vi "OCT OpenCL.vi"() -> ()   [LabVIEW 2014]
doc: "I. Description:\nThis example demonstrates how to acquire a continuous amount of data (Waveform) using the DAQ device's internal clock.\n\nII. Instructions for Running:\n1. Create an analog input voltage channel.\n2. Set the rate for the sample clock. Additionally, define the sample mode to be continuous.\n3. Call the Start VI to start the acquisition.\n4. Read the waveform data in a loop until the user hits the stop button or an error occurs.\nNote: This example reads data from one or more channels and returns an array of data. Use the Index Array function to access an individual channel of data.\n5. Call the Clear Task VI to clear the Task.\n6. Use the popup dialog box to display an error if any.\n\nIV. I/O Connections Overview:\nMake sure your signal input terminal matches the Physical Channel I/O Control. For further connection information, refer to your hardware reference manual."
uses:
  ATS-VI/ATS_ctl/Device_Ctrl.ctl
  ATS-VI/ATS_ctl/ATS_Async_Ctrl.ctl
  ATS-VI/ATS_ctl/ATS_Async_Mode.ctl
  ATS-VI/ATS_ctl/ATS_DMA_Channel.ctl
  ATS-VI/ATS_ctl/ATS_ReadSamples.ctl
  ATS-VI/ATS_ctl/ATS_Check_Ctrl.ctl
  ATS-VI/ATS_ctl/ClockSource.ctl
  Galvo VIs/galvo_states.ctl
  Signal Processing/processing_states.ctl
  En Face/En Face States.ctl
  Saving Data/Saving Data States.ctl
  Type Defs/OCT Hardware States.ctl
  ATS-VI/ATS_ctl/Range.ctl
  ATS-VI/ATS_ctl/Impedance.ctl
  Type Defs/OCT Imaging Parameters Cluster.ctl
  Signal Processing/Display Raw Data states.ctl
  ATS-VI/ATS_ctl/Record.ctl
  ATS-VI/ATS_ctl/ClockRate.ctl
  ATS-VI/ATS_ctl/ClockEdge.ctl
  ATS-VI/ATS_ctl/Clock.ctl
  ATS-VI/ATS_ctl/Coupling.ctl
  ATS-VI/ATS_ctl/Bandwidth.ctl
  ATS-VI/ATS_ctl/InputCtrl.ctl
  ATS-VI/ATS_ctl/TriggerOperation.ctl
  ATS-VI/ATS_ctl/TriggerEngine.ctl
  ATS-VI/ATS_ctl/ExtTrigRange.ctl
  ATS-VI/ATS_ctl/ExtTrigger.ctl
  ATS-VI/ATS_ctl/Trigger.ctl
  ATS-VI/ATS_ctl/ATS_Global.ctl
  OpenCL/OpenCL States.ctl
  <vilib>/RaptorView/OpenCLV/User Controls/Array Dimensions.ctl
  DAQ Status States.ctl
  Type Defs/Display States.ctl
  ATS-VI/ATS_ctl/ATS_Async_Setting.ctl
  Type Defs/OCT DAQ Channel Data Type.ctl
panel:
  out "Background Array":u16[](array[numeric])
  in  "Calibrate":bool
  in  "Save Sweep Button":bool
  in  "Linear?":bool
  in  "Data Format":T1
  out "BScan":sgl[][](graph)
  in  "Display":T2
  in  "Save Sweep":bool
  in  "Stop Button":bool
  in  "B-Scans Per Buffer":i32=1
  out "Current State":T3
  in  "Channels":tag="Dev2/ao0:1"
  in  "Trigger Source":tag="/Dev2/PFI7"
  in  "Imaging Parameters":T4={"Points Per A-Scan"=0, "A-Scans per B-Scan"=0, "Voltage Range"=1.0, "Card Resolution (bits)"=12}
  out "First Time?":bool=TRUE
  out "Save Data":bool
  in  "Async_Setting":T5
  out "Processing Finished":bool
  in  "OCT Hardware States":T3=enum."Initialize DAQ"
  out "Save State":T6=enum."Do Nothing"
  out "Clock Length":u32=9184
  out "Reset DAQ":bool
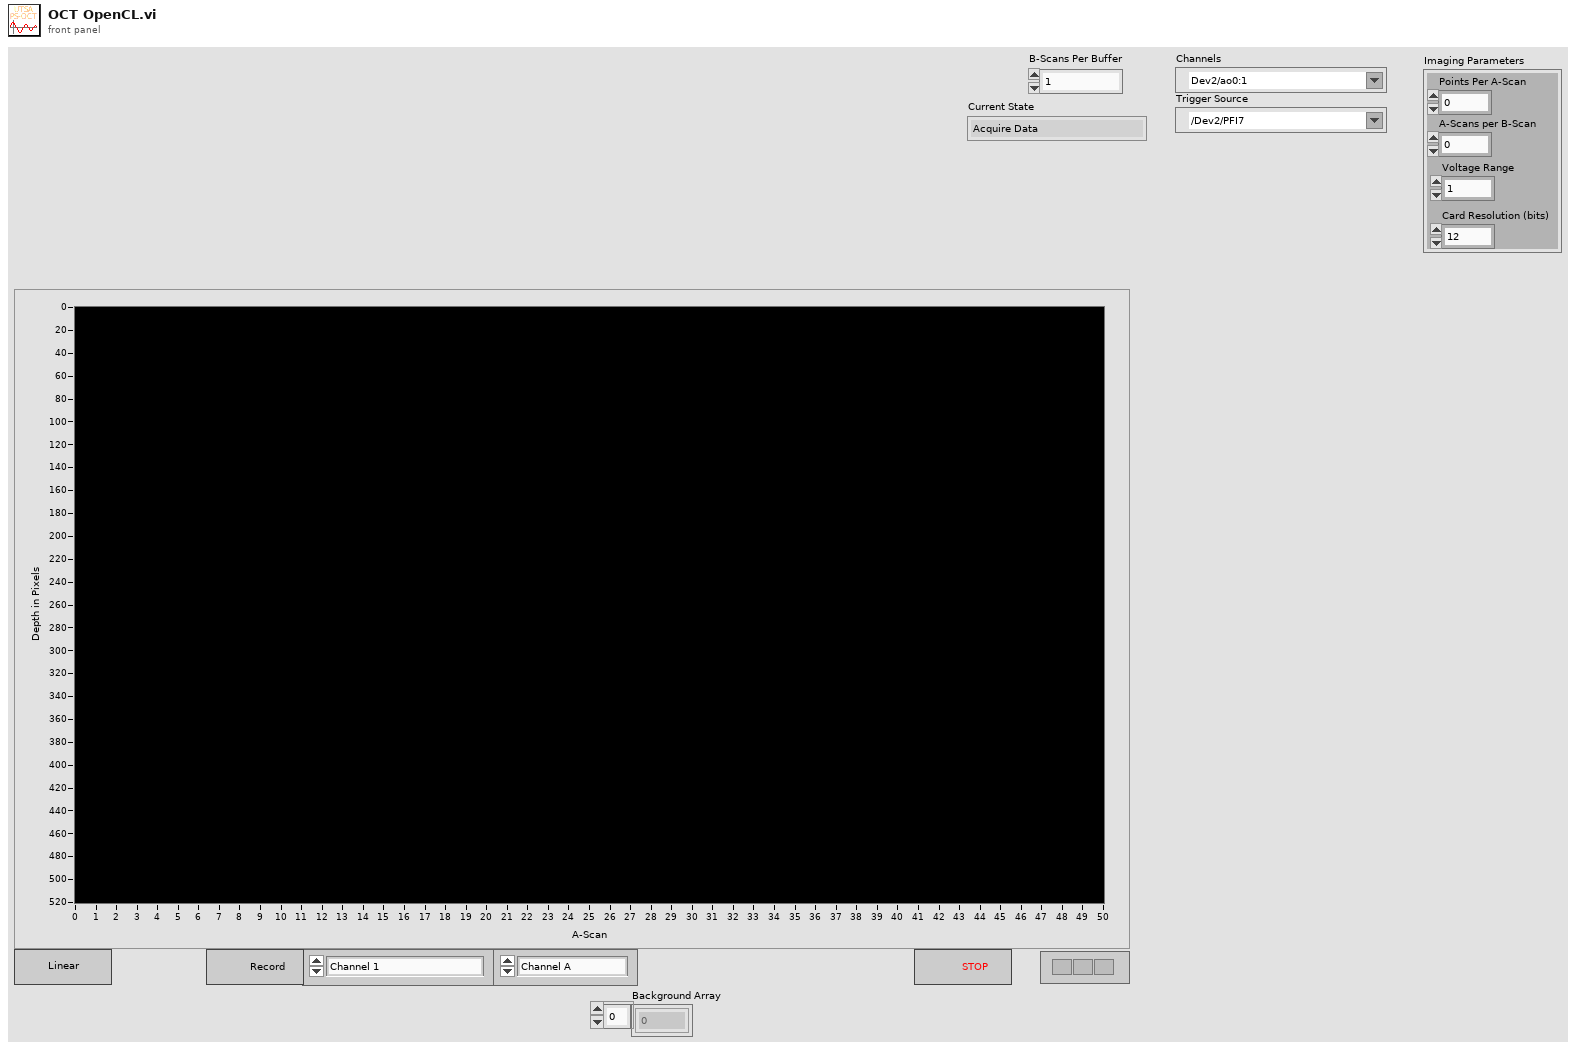
[diagram p1: front panel]
types:
  T1 = typedef "OCT DAQ Channel Data Type.ctl" = enum16{"Channel 1", "Channel 2", "Channel 1 and 2"}
  T2 = typedef "Display States.ctl" = enum16{"Channel A", "Channel B"}
  T3 = typedef "OCT Hardware States.ctl" = enum16{"Acquire Data", "Initialize Laser", "Initialize Galvos", "Startup", "Reset DAQ", "Background Subtraction", "Acquire Background", "Update DAQ Parameters", "Stop", "Set Clock", "Initialize DAQ", "Set Resampling Array", "Save Sweep", "Configure Laser"}
  T4 = typedef "OCT Imaging Parameters Cluster.ctl" = cluster{"Points Per A-Scan":i32, "A-Scans per B-Scan":i32, "Voltage Range":sgl, "Card Resolution (bits)":u16}
  T5 = typedef "ATS_Async_Setting.ctl" = cluster{"UseHeader":u32, "Rec/Buffer":u32, "Total_Rec":u32, "DataBuffer":bool, "GetProcessedData":bool}
  T6 = typedef "Saving Data States.ctl" = enum16{"Get Queue Size", "Get Queue", "Get Timeout", "Flush Queue", "Close Files", "Create Files", "Do Nothing", "Initialize", "Enqueue Data", "Save Data", "Shutdown"}
  T7 = typedef "ATS_Global.ctl" = cluster{"Record":T8, "Clock":T9, "Input A":T13, "Input B":T13, "Trigger":T18}
  T8 = typedef "Record.ctl" = cluster{"Count":u32, "Presize":u32, "Length":u32}
  T9 = typedef "Clock.ctl" = cluster{"ClckSource":T10, "ClckRate":T11, "ClckEdge":T12, "Decimation":u32}
  T10 = typedef "ClockSource.ctl" = enum16{"Internal", "External", "Medium Ext.", "Slow Ext.", "Ext. AC", "Ext. DC", "Ext. (PLL)"}
  T11 = typedef "ClockRate.ctl" = u32
  T12 = typedef "ClockEdge.ctl" = u16
  T13 = typedef "InputCtrl.ctl" = cluster{"Coupling":T14, "Range":T15, "Impedance":T16, "Bandwidth":T17}
  T14 = typedef "Coupling.ctl" = enum16{"AC", "DC"}
  T15 = typedef "Range.ctl" = u32
  T16 = typedef "Impedance.ctl" = enum16{"1M ohms", "50 ohms"}
  T17 = typedef "Bandwidth.ctl" = enum16{"Full Bandwidth", "Reduce Bandwidth"}
  T18 = typedef "Trigger.ctl" = cluster{"TrigOperation":T19, "Timeout (s)":dbl, "Trig. Delay":u32, "Engine X":T20, "Engine Y":T20, "ExtTrigControl":T21}
  T19 = typedef "TriggerOperation.ctl" = enum16{"Only X", "Only Y", "X or Y", "X and Y", "X xor Y", "X and not Y", "not X and Y"}
  T20 = typedef "TriggerEngine.ctl" = cluster{"Source":enum32{"Chan_A", "Chan_B", "External", "Disable"}, "Slope":enum32{"Positive", "Negative"}, "Level":u32}
  T21 = typedef "ExtTrigger.ctl" = cluster{"Coupling":T14, "Range":T22}
  T22 = typedef "ExtTrigRange.ctl" = enum16{"1 V", "5 V", "TTL"}
  T23 = typedef "galvo_states.ctl" = enum16{"Reset", "Reset Galvos?", "Center Galvos", "Register Callback", "Get Scan Parameters", "Show", "Initialize", "Run Raster", "Load Raster", "Run Circle", "Shutdown"}
  T24 = typedef "OpenCL States.ctl" = enum16{"Allocate Memory", "Get U16 Memory Dimension", "Compile Kernels", "Create Device", "Write", "Read", "Operate", "Delete Memory", "Delete"}
  T25 = typedef "processing_states.ctl" = enum16{"Initialize", "Set Background", "Update Imaging Parameters", "Get Queue", "Process Data", "Get Size", "Flush Data", "Set Reample Array", "Get Last Processed BScan", "Shutdown"}
  T26 = typedef "En Face States.ctl" = enum16{"Save BMP", "Show", "Clear En Face", "Update EnFace"}
  T27 = typedef "Galvo.lvclass/Scanning Cluster.ctl" = cluster{"Fast Axis Offset":sgl, "Slow Axis Offset":sgl, "Slow Axis Amp":sgl, "Fast Axis Amp":sgl, "Scan Pattern":enum16{"Raster"}}
  T28 = typedef "Processed OCT Data.ctl" = cluster{"Intensity A":sgl[][][], "Intensity B":sgl[][][]}
  T29 = typedef "ATS_Async_Ctrl.ctl" = enum16{"SetupDMA", "StartCapture", "Get", "Get_Stream", "Abort", "Stop"}
  T30 = typedef "ATS_ReadSamples.ctl" = cluster{"Offset":i32, "Length":u32}
  T31 = typedef "ATS_DMA_Channel.ctl" = enum16{"Channel_A", "Channel_B", "A & B"}
  T32 = typedef "ATS_Async_Mode.ctl" = enum16{"Continuous", "Triggered", "No-Pre-Trigger", "Traditional"}
  T33 = typedef "ATS_Check_Ctrl.ctl" = enum16{"None", "NO_ATS9462", "ATS9462_Traditional", "Verify Board", "OnBoard Memory", "Board & Memory", "Master/Slave", "NO Master/Slave"}
  T34 = typedef "Device_Ctrl.ctl" = enum16{"Status", "About", "Arm", "ForceTrig", "Abort", "Initialize", "Init (NoPreset)", "Info", "Close", "Calibrate", "SetManually", "LED_ON", "LED_OFF"}
  T35 = typedef "DAQ Status States.ctl" = enum16{"Get", "Show"}
  T36 = typedef "Display Raw Data states.ctl" = enum16{"Add Raw", "Add Processed", "Show"}
  T37 = typedef "Array Dimensions.ctl" = cluster{"Depth":u64, "Height":u64, "Width":u64}
  T38 = typedef "ATS_Async_Status.ctl" = cluster{"Start DMA":bool, "StartCapture":bool, "Valid":bool, "Completed":bool, "InProgress":bool, "Timeout":bool, "Overflow":bool, "Error":bool}
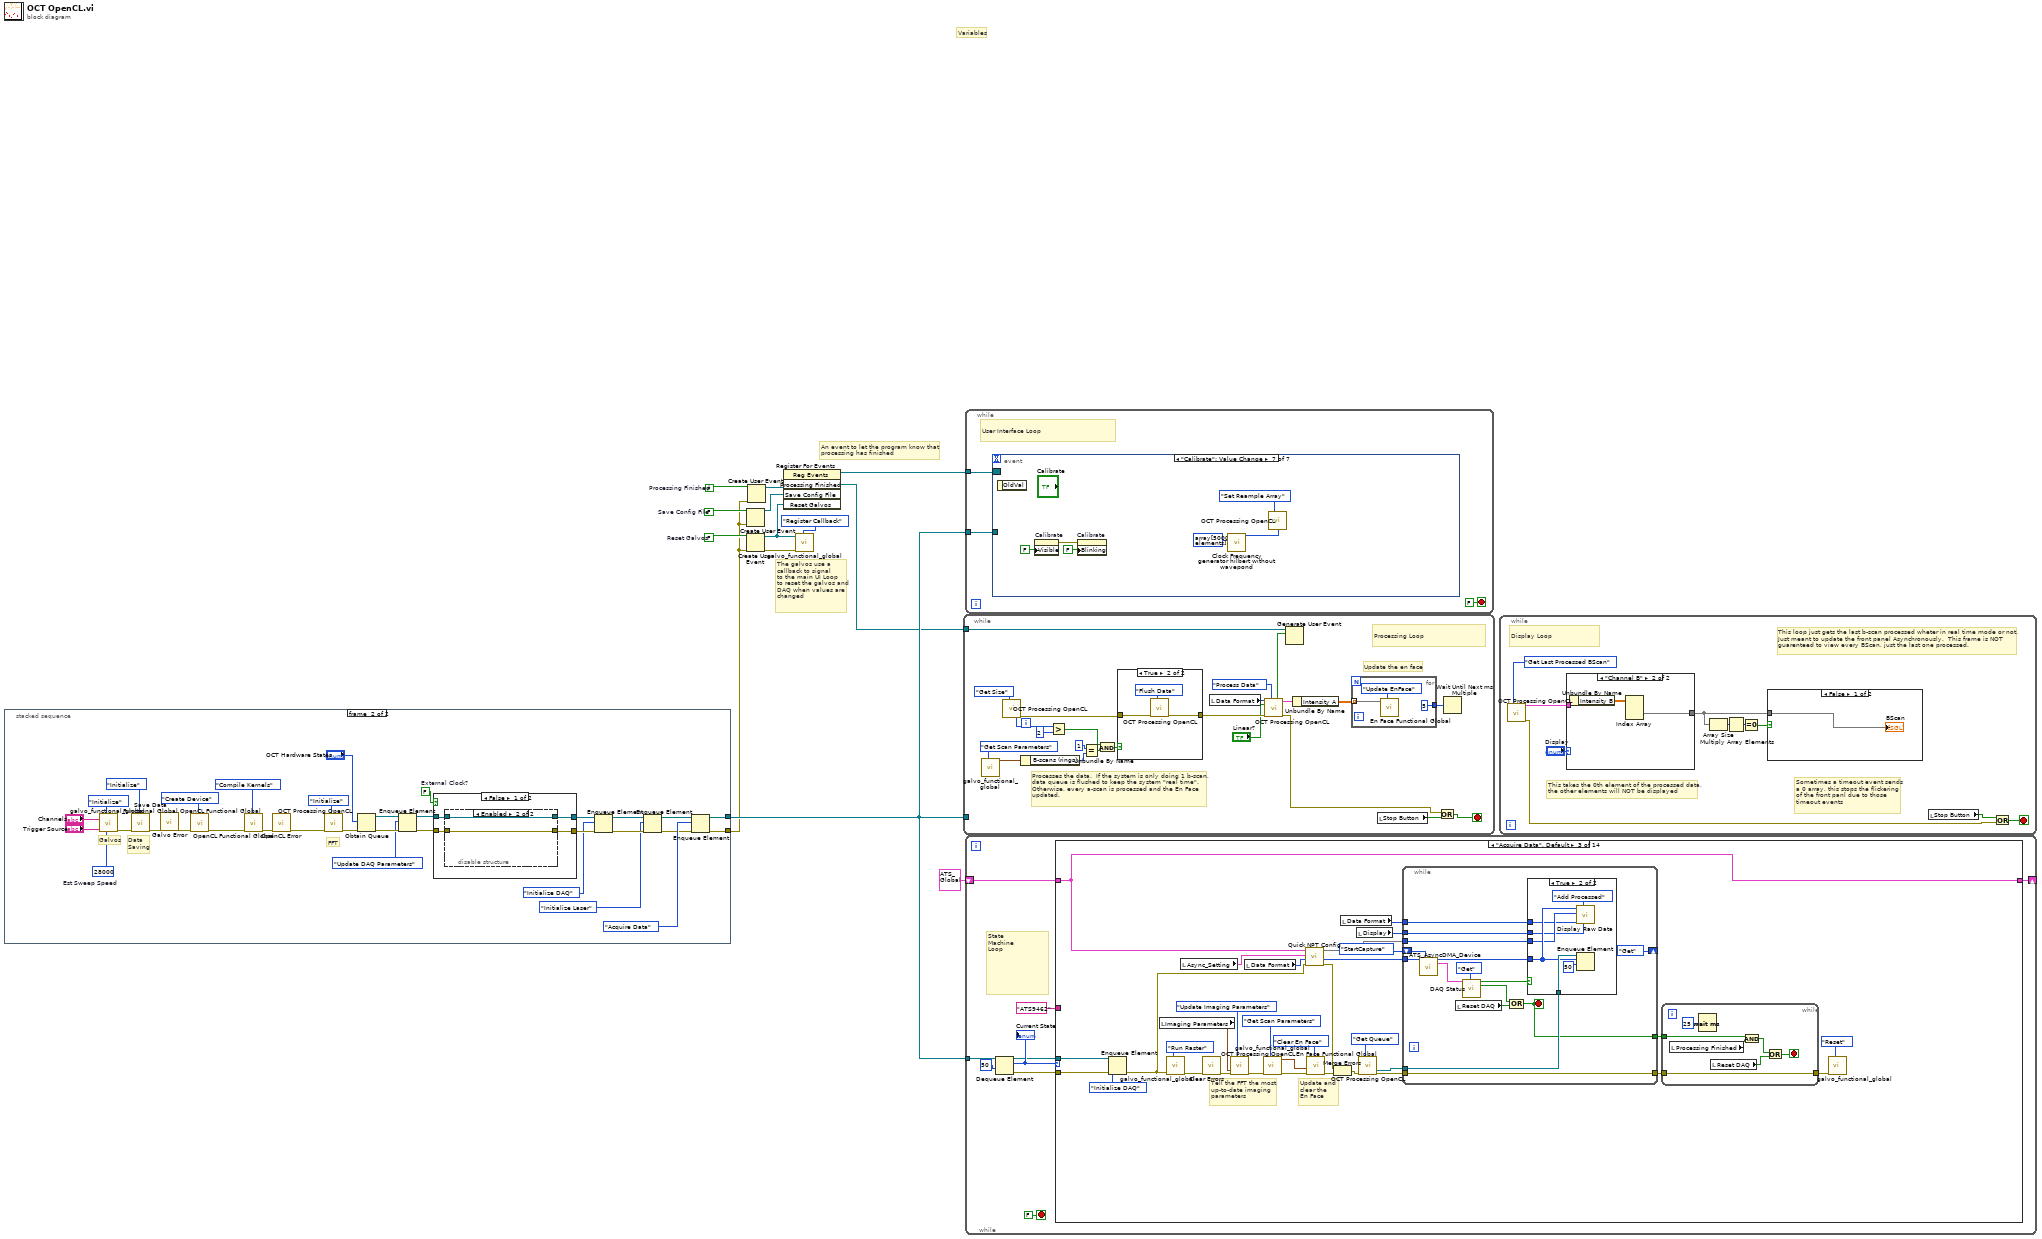
[diagram p0: block diagram]
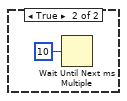
[diagram p3: hidden frame]
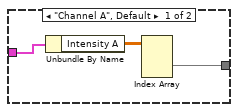
[diagram p4: hidden frame]
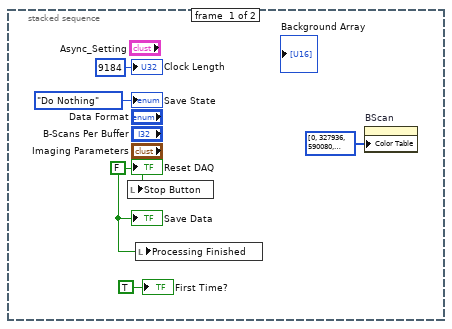
[diagram p5: hidden frame]
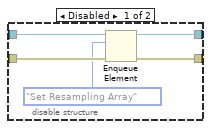
[diagram p6: hidden frame]
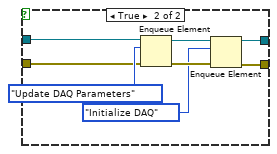
[diagram p7: hidden frame]
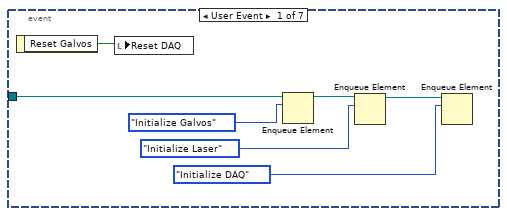
[diagram p8: hidden frame]
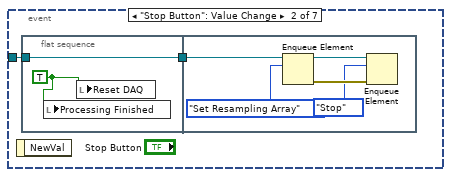
[diagram p9: hidden frame]
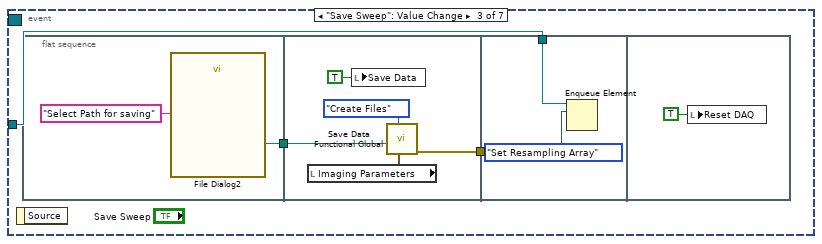
[diagram p10: hidden frame]
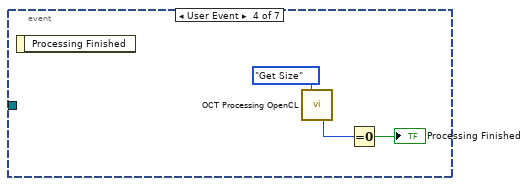
[diagram p11: hidden frame]
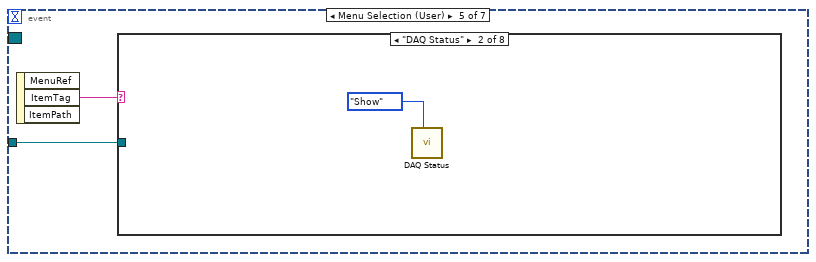
[diagram p12: hidden frame]
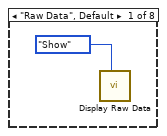
[diagram p13: hidden frame]
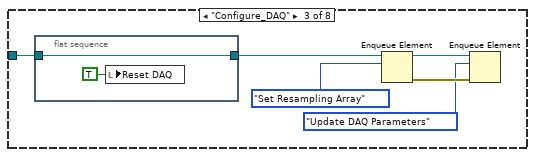
[diagram p14: hidden frame]
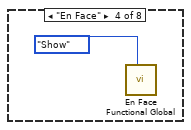
[diagram p15: hidden frame]
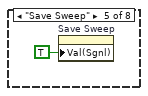
[diagram p16: hidden frame]
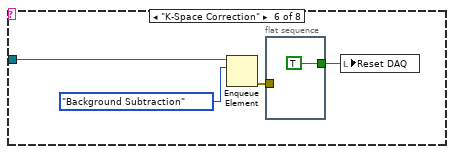
[diagram p17: hidden frame]
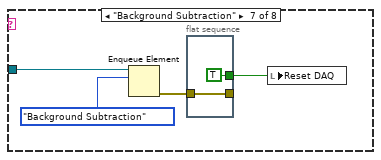
[diagram p18: hidden frame]
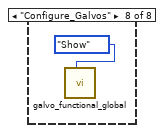
[diagram p19: hidden frame]
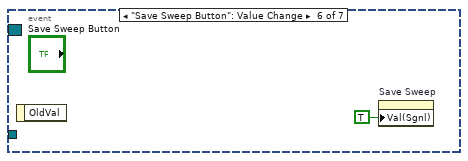
[diagram p20: hidden frame]
diagram:
  w6 = FALSE  # Reset Galvos
  w9 = FALSE  # Save Config File
  w12 = FALSE  # Processing Finished
  # "The galvos use a \ncallback to signal\nto the main UI Loop\nto reset the galvos and\nDAQ when values are\nchanged"
  # "An event to let the program know that\nprocessing has finished"
  # "Variables"
  n1 = stacked-sequence {
    tunnel: [_ w34] -> w10
    tunnel: [_ w33] -> w1
    frame #0 {
      w14 = FALSE ("Sweep Ready for saving")
      n2 = local write "Stop Button"(w14) -> ()
      n3 = local write "Processing Finished"(w14) -> ()
      n4 = property on="BScan" class="IntGraph (strict)"("Color Table"=u32[] [0, 327936, 590080, 852224, 983296, 1114624, 1180160, 1311232, 1442304, 1573632, 1704704, 1770240, 1901312, 1966848, 2098176, 2163712, 2294784, 2491392, 2557184, 2688256, 2753792, 2884864, 2950656, 3081728, 3147264, 3344129, 3475457, 3540993, 3672321, 3738113, 3869185, 3934977, 4066305, 4197633, 4328961, 4394497, 4460289, 4591617, 4657409, 4788481, 4854273, 4985601, 5116929, 5248257, 5314049, 5379841, 5511169, 5576961, 5708033, 5773825, 5905153, 6036482, 6167810, 6233346, 6299138, 6430466, 6496258, 6562050, 6693634, 6759426, 6890754, 7022082, 7087874, 7153666, 7284994, 7350786, 7482114, 7547906, 7613698, 7745026, 7876354, 8007682, 8073474, 8139522, 8205314, 8336642, 8467970, 8533763, 8599555, 8665347, 8731139, 8862467, 8993795, 9059587, 9125380, 9191428, 9257220, 9388548, 9454340, 9520132, 9585924, 9717253, 9848837, 9914629, 9980165, 10045957, 10177541, 10243334, 10309126, 10375174, 10440966, 10572294, 10703623, 10769416, 10835208, 10901256, 10967049, 11033097, 11033609, 11099401, 11165450, 11231242, 11231754, 11297547, 11363339, 11429131, 11495180, 11495692, 11561740, 11693069, 11758861, 11759373, 11825165, 11891214, 11957006, 12022799, 12023311, 12089103, 12220944, 12286736, 12286736, 12352529, 12418577, 12484370, 12550162, 12615954, 12681747, 12747796, 12813588, 12813845, 12879894, 12945686, 13077015, 13142808, 13143064, 13208856, 13274905, 13340697, 13340953, 13472282, 13538075, 13604379, 13670172, 13735964, 13801757, 13867550, 13933343, 13999392, 13999648, 14065441, 14131234, 14197027, 14197541, 14263334, 14329383, 14395176, 14460969, 14592553, 14658346, 14724139, 14789932, 14790189, 14856238, 14922287, 14988080, 15053873, 15054130, 15119923, 15185972, 15251765, 15317559, 15383353, 15449146, 15449660, 15515454, 15515968, 15516226, 15582021, 15582278, 15582536, 15648587, 15648844, 15714639, 15714897, 15715155, 15780949, 15781463, 15847256, 15847770, 15848028, 15913823, 15914081, 15979875, 15980133, 15980391, 16046441, 16046444, 16046703, 16046705, 16112500, 16113015, 16113274, 16113277, 16179072, 16179330, 16179588, 16245384, 16245387, 16245389, 16245648, 16311443, 16376982, 16377241, 16377499, 16443294, 16443553, 16443555, 16443815, 16509866, 16510124, 16510127, 16575923, 16575924, 16576182, 16576441, 16576443, 16576702, 16576705, 16576963, 16577222, 16577224, 16577482, 16577485, 16577743, 16577745, 16578004, 16578262, 16578264, 16578523, 16578782, 16579040, 16579299, 16579301, 16579303, 16579562, 16579821]) -> ()  [unwired: 2 in, 2 out]
      "Clock Length" <- u32 9184 ("Clock Length")
      "Save State" <- Saving_Data_States."Do Nothing" ("Save State")
      "Reset DAQ" <- w14
      "Save Data" <- w14
      "First Time?" <- TRUE ("First Time?")
    }
    frame #1 {
      w38 = 28000  # Est Sweep Speed
      w39 = FALSE  # External Clock?
      # "FFT"
      # "Data \nSaving"
      # "Galvos"
      n5 = call "galvo_functional_global.vi"("Est Sweep Speed"=w38, "State"=galvo_states."Initialize", "Trigger Source"="Trigger Source", "Analog Output"="Channels") -> ("error out"=w43:errorcluster)  [unwired: 6 in, 1 out]
      n6 = call "Save Data Functional Global.vi"("States"=Saving_Data_States."Initialize", "error in (no error)"=w43) -> ("error out"=w21:errorcluster)  [unwired: 6 in, 3 out]
      n7 = call "Galvo Error.vi"("error in (no error)"=w21) -> ("error out"=w20:errorcluster)  [unwired: 10 in]
      n8 = call "OpenCL Functional Global.vi"("States"=OpenCL_States."Create Device", "Error In"=w20) -> ("Error Out"=w23:errorcluster)  [unwired: 6 in, 3 out]
      n9 = call "OpenCL Functional Global.vi"("States"=OpenCL_States."Compile Kernels", "Error In"=w23) -> ("Error Out"=w19:errorcluster)  [unwired: 6 in, 3 out]
      n10 = call "OpenCL Error.vi"("error in (no error)"=w19) -> ("error out"=w18:errorcluster)  [unwired: 10 in]
      n11 = call "OCT Processing OpenCL.vi"("State"=processing_states."Initialize", "error in (no error)"=w18) -> ("error out"=w46:errorcluster)  [unwired: 9 in, 4 out]
      n12 = Obtain Queue(element data type="OCT Hardware States", error in (no error)=w46) -> (queue out=w36:refnum<queue>, error out=w37:errorcluster)  [unwired: 3 in, 1 out]
      n13 = Enqueue Element(queue=w36, element=OCT_Hardware_States."Update DAQ Parameters", error in (no error)=w37) -> (queue out=w30:refnum<queue>, error out=w29:errorcluster)  [unwired: 1 in, 1 out]
      n14 = case shown="False" w39 {
        tunnel: [w51 w67] -> w50
        tunnel: [w52 w66] -> w49
        tunnel: w30 -> [w54 w63]
        tunnel: w29 -> [w53 w62]
        frame False {
          n15 = disable-structure shown="Enabled" {
            disable-tunnel: w54 -> [w59 w61]
            disable-tunnel: w53 -> [w58 w60]
            disable-tunnel: [w57 w60] -> w52
            disable-tunnel: [w56 w61] -> w51
            frame Disabled {
              n16 = Enqueue Element(queue=w59, element=OCT_Hardware_States."Set Resampling Array", error in (no error)=w58) -> (queue out=w56:refnum<queue>, error out=w57:errorcluster)  [unwired: 1 in, 1 out]
            }
            frame Enabled {
            }
          }
        }
        frame True {
          n17 = Enqueue Element(queue=w63, element=OCT_Hardware_States."Update DAQ Parameters", error in (no error)=w62) -> (queue out=w69:refnum<queue>, error out=w68:errorcluster)  [unwired: 1 in, 1 out]
          n18 = Enqueue Element(queue=w69, element=OCT_Hardware_States."Initialize DAQ", error in (no error)=w68) -> (queue out=w67:refnum<queue>, error out=w66:errorcluster)  [unwired: 1 in, 1 out]
        }
      }
      n19 = Enqueue Element(queue=w50, element=OCT_Hardware_States."Initialize DAQ", error in (no error)=w49) -> (queue out=w28:refnum<queue>, error out=w25:errorcluster)  [unwired: 1 in, 1 out]
      n20 = Enqueue Element(queue=w28, element=OCT_Hardware_States."Initialize Laser", error in (no error)=w25) -> (queue out=w27:refnum<queue>, error out=w26:errorcluster)  [unwired: 1 in, 1 out]
      n21 = Enqueue Element(queue=w27, element=OCT_Hardware_States."Acquire Data", error in (no error)=w26) -> (queue out=w34:refnum<queue>, error out=w33:errorcluster)  [unwired: 1 in, 1 out]
    }
  }
  n22 = Create User Event(user event datatype=w9, error in=w1) -> (user event=w8:refnum<user-event>)  [unwired: 1 out]
  n23 = Create User Event(user event datatype=w6, error in=w1) -> (user event=w5:refnum<user-event>, error out=w2:errorcluster)
  n24 = Create User Event(user event datatype=w12, error in=w1) -> (user event=w7:refnum<user-event>)  [unwired: 1 out]
  n25 = register-events(w7, w8, w5) -> (reference out=w11:refnum<event-registration>)  [unwired: 2 in, 1 out]
  n26 = call "galvo_functional_global.vi"("State"=galvo_states."Register Callback", "error in (no error)"=w2, "user event out"=w5) -> ()  [unwired: 7 in, 2 out]
  n27 = while {
    tunnel: w7 -> [w83]
    tunnel: w10 -> [_]
    stop <- w71 stop-if-true
    # "Processing Loop"
    # "Update the en face"
    # "Processes the data.  If the system is only doing 1 b-scan, \ndata queue is flushed to keep the system \"real time\".\nOtherwise, every a-scan is processed and the En Face\nupdated."
    n28 = call "galvo_functional_global.vi"("State"=galvo_states."Get Scan Parameters") -> ("Scanning Output"=w76:T27)  [unwired: 9 in, 1 out]
    n29 = call "OCT Processing OpenCL.vi"("State"=processing_states."Get Size") -> ("# elements in queue"=w89:i32, "error out"=w80:errorcluster)  [unwired: 10 in, 3 out]
    n30 = Unbundle By Name(w76) -> ("B-scans (rings)"=w85:u32)
    n31 = Greater?(x=w89, y=2) -> (0:w90:bool)
    n32 = Equal?(x=u32 1, y=w85) -> (x = y?=w77:bool)
    n33 = And(x=w90, y=w77) -> (x .and. y?=w78:bool)
    n34 = case shown="True" w78 {
      tunnel: w80 -> [w96 w99]
      tunnel: [w96 w98] -> w79
      frame False {
      }
      frame True {
        n35 = call "OCT Processing OpenCL.vi"("State"=processing_states."Flush Data", "error in (no error)"=w99) -> ("error out"=w98:errorcluster)  [unwired: 9 in, 4 out]
      }
    }
    n36 = local read "Data Format"() -> (w84:T1)
    n37 = call "OCT Processing OpenCL.vi"("Data Format"=w84, "State"=processing_states."Process Data", "Linear?"="Linear?", "error in (no error)"=w79) -> ("Time Out"=w82:bool, "Processed OCT Data"=w87:T28, "error out"=w70:errorcluster)  [unwired: 7 in, 2 out]
    n38 = Generate User Event(user event=w83, event data cluster=w82) -> ()  [unwired: 2 in, 2 out]
    n39 = Unbundle By Name(w87) -> ("Intensity A"=w81:sgl[][][])
    n40 = for {
      tunnel: w81 -> [w94] mode=indexing
      tunnel: [u32 5 ("millisecond multiple")] -> w74
      n41 = call "En Face Functional Global.vi"(7:En_Face_States."Update EnFace" ("En Face States"), "Intensity Graph 2"=w94) -> ()  [unwired: 8 in, 2 out]
    }
    n42 = local read "Stop Button"() -> (w72:bool)
    n43 = Or(x=w70, y=w72) -> (x .or. y?=w71:bool)
    n44 = Wait Until Next ms Multiple(millisecond multiple=w74) -> ()  [unwired: 1 out]
  }
  n45 = while {
    tunnel: w10 -> [w108]
    shift-right: [w102] -> _
    shift-left: T7 {"Record"={"Count"=0, "Presize"=0, "Length"=0}, "Clock"={"ClckSource"=enum."Internal", "ClckRate"=0, "ClckEdge"=0, "Decimation"=0}, "Input A"={"Coupling"=enum."DC", "Range"=12, "Impedance"=enum."1M ohms", "Bandwidth"=enum."Full Bandwidth"}, "Input B"={"Coupling"=enum."DC", "Range"=12, "Impedance"=enum."1M ohms", "Bandwidth"=enum."Full Bandwidth"}, "Trigger"={"TrigOperation"=enum."Only X", "Timeout (s)"=-1.0, "Trig. Delay"=0, "Engine X"={"Source"=enum."Chan_A", "Slope"=enum."Positive", "Level"=0}, "Engine Y"={"Source"=enum."Chan_A", "Slope"=enum."Positive", "Level"=0}, "ExtTrigControl"={"Coupling"=enum."AC", "Range"=enum."1 V"}}} ("Value") -> [w101]
    stop <- FALSE stop-if-true
    # "State\nMachine\nLoop"
    n46 = Dequeue Element(queue=w108, timeout in ms (-1)=50) -> (queue out=w104:refnum<queue>, element=w106:T3, error out=w105:errorcluster)  [unwired: 1 in, 1 out]
    "Current State" <- w106
    n47 = case shown="\"Acquire Data\", Default" w106 {
      tunnel: w105 -> [_ w155 w212 w272 w326 _ w391 _ _ _ w429 w437 w455 w461]
      tunnel: w104 -> [_ _ w213 w271 w340 _ w392 _ _ _ w430 w435 _ _]
      tunnel: "ATS9462" ("BoardToVerify") -> [_ w169 _ _ _ _ _ w399 _ _ _ _ _ _]
      tunnel: [w109 w163 w231 w283 w315 w377 w384 w398 w414 w415 w425 w439 w448 w459] -> w102
      tunnel: w101 -> [w109 w162 w231 w283 w315 w377 w384 w398 w414 _ w425 w439 w448 w459]
      frame "Initialize DAQ" {
        # "Gage if you need\nthe gage card,\nenable here"
        n48 = case shown="True" FALSE {
          tunnel: w109 -> [_ w111]
          frame False {
          }
          frame True {
            w115 = 0 ("DeviceIn")
            n49 = local read "Clock Length"() -> (w117:u32)
            n50 = local read "Async_Setting"() -> (w113:T5)
            n51 = Bundle By Name(cluster=w113, "UseHeader"=u32 0, "Rec/Buffer"=u32 125, "Total_Rec"=u32 0) -> (w114:T5)
            n52 = Unbundle By Name(w111) -> ("Record.Presize"=w118:u32)
            n53 = Bundle By Name(cluster=T30 {"Offset"=0, "Length"=0} ("ReadSamples"), "Length"=w117, "Offset"=w118) -> (w116:T30)
            n54 = call "ATS_AsyncDMA_Device.vi"("DeviceIn"=w115, "ATS_Async_Ctrl"=ATS_Async_Ctrl."SetupDMA" ("ATS_DMA_Ctrl"), "Async_Mode"=ATS_Async_Mode."Traditional", "Async_Setting"=w114, "Channel"=ATS_DMA_Channel."Channel_B", "ReadSamples"=w116, "Start Now / Wait"=TRUE) -> ("Buffer"=w123:u16[])  [unwired: 4 in, 4 out]
            n55 = while {
              tunnel: w123 -> [_]
              shift-right: [ATS_Async_Ctrl."Get" ("ATS_Async_Ctrl")] -> _
              shift-left: ATS_Async_Ctrl."StartCapture" ("ATS_Async_Ctrl") -> [w137]
              tunnel: w115 -> [w131]
              stop <- w134 stop-if-true
              n56 = call "ATS_AsyncDMA_Device.vi"("DeviceIn"=w131, "ATS_Async_Ctrl"=w137) -> ("Buffer"=w129:u16[], "Async_Status"=w128:T38)  [unwired: 9 in, 3 out]
              n57 = Unbundle By Name(w128) -> ("Valid"=w130:bool, "Completed"=w139:bool, "Start DMA"=w140:bool, "Timeout"=w141:bool, "Error"=w138:bool)
              n58 = property on="Reset DAQ" class="Bool (strict)"() -> ("Value"=w135:bool)  [unwired: 2 in, 2 out]
              n59 = local read "Clock Length"() -> (w132:u32)
              n60 = Compound Arithmetic op=OR(w139, invert w140, w141, w138, w135) -> (w133:bool)
              n61 = case shown="True" w130 {
                selector: w130 -> [w142 w145]
                tunnel: w129 -> [_ w144]
                tunnel: [w142 w145] -> w134
                tunnel: w133 -> [_ _]
                tunnel: w132 -> [_ w143]
                frame False {
                }
                frame True {
                  n62 = Array Subset(array=w144, length=w143) -> (w146:u16[])  [unwired: 1 in]
                  n63 = call "Clock Frequency generator hilbert.vi"(7:6300.0 ("Sweep Speed"), "Acquisition speed (S/s)"=180000000.0 ("Sweep Speed"), "k-space signal in"=w146, "number of frequency updates"=4385) -> ("Error Out"=w151:errorcluster, "frequency\nsteps"=w150:i32)  [unwired: 6 in]
                  n64 = call "wavepond sequence.vi"("Error In"=w151, "Number of updates"=w150) -> ()  [unwired: 9 in, 1 out]
                }
              }
            }
          }
        }
      }
      frame "Initialize DAQ" {
        # "B-Scans per buffer should be around 4 if \ntaking more than 1 to minimize data transfer"
        # "If B Scans is 1, set total records to 0,\notherwise it should be A-Scans Per\nBScan times BScans"
        # "BScans Per Buffer"
        n65 = local read "First Time?"() -> (w166:bool)
        n66 = case shown="True" w166 {
          tunnel: [w195 w205] -> w191
          tunnel: w169 -> [_ w201]
          tunnel: [FALSE ("First Time?") FALSE ("First Time?")] -> w165
          frame False {
            n67 = flat-sequence {
              tunnel: [w197] -> w195
              frame #0 {
                w197 = 0 ("DeviceIn")
                n68 = call "ATS_AsyncDMA_Device.vi"("DeviceIn"=w197, "ATS_Async_Ctrl"=ATS_Async_Ctrl."Stop") -> ("ReadSamples_Out"=w200:T30)  [unwired: 9 in, 4 out]
                n69 = call "ATS_AsyncDMA_Device.vi"("DeviceIn"=w197, "ATS_Async_Ctrl"=ATS_Async_Ctrl."Abort", "ReadSamples"=w200) -> ()  [unwired: 8 in, 5 out]
              }
            }
          }
          frame True {
            n70 = call "ATS_Device.vi"("BoardToVerify"=w201, "ATS_Check"=ATS_Check_Ctrl."Verify Board", "DevCtrl"=Device_Ctrl."Initialize", "DeviceIn"=0 ("Device")) -> ("error out"=w203:errorcluster, "DeviceOut"=w207:i32)  [unwired: 1 in, 5 out]
            n71 = call "ATS_Device.vi"("error in (no error)"=w203, "DevCtrl"=Device_Ctrl."Abort", "DeviceIn"=w207) -> ("DeviceOut"=w205:i32)  [unwired: 2 in, 6 out]
          }
        }
        n72 = flat-sequence {
          tunnel: w155 -> [w193]
          tunnel: [w193] -> w156
          frame #0 {
            n73 = local write "Processing Finished"(FALSE ("Reset DAQ")) -> ()
            n74 = local write "Reset DAQ"(FALSE ("Reset DAQ")) -> ()
          }
        }
        n75 = call "Save Data Functional Global.vi"("States"=Saving_Data_States."Flush Queue", "error in (no error)"=w156) -> ("error out"=w158:errorcluster)  [unwired: 6 in, 3 out]
        n76 = call "OCT Processing OpenCL.vi"("State"=processing_states."Flush Data", "error in (no error)"=w158) -> ("error out"=w154:errorcluster)  [unwired: 9 in, 4 out]
        n77 = local write "First Time?"(w165) -> ()
        n78 = Unbundle By Name(w162) -> ("Record.Length"=w170:u32)
        n79 = call "ATS_MS_Set_Device.vi"("Set_Manually (F)"=FALSE, "Setup_In"=w162, "DeviceIn"=w191) -> ("Setup_Out"=w163:T7)  [unwired: 3 in, 5 out]
        n80 = call "galvo_functional_global.vi"("State"=galvo_states."Get Scan Parameters", "error in (no error)"=w154) -> ("Scanning Output"=w161:T27)  [unwired: 8 in, 1 out]
        n81 = Unbundle By Name(w161) -> ("B-scans (rings)"=w176:u32, "A(cluster)/B"=w186:u32, "B-scans (rings)"=w181:u32, "A(cluster)/B"=w180:u32, "B-scans (rings)"=w178:u32, "A(cluster)/B"=w172:u32)
        n82 = local read "Async_Setting"() -> (w168:T5)
        n83 = Not Equal?(x=w178, y=u32 1 ("x")) -> (x != y?=w179:bool)
        n84 = Equal?(x=u32 1, y=w176) -> (x = y?=w182:bool)
        n85 = local read "B-Scans Per Buffer"() -> (w164:i32)
        n86 = Select(t=u32 4 ("y"), s=w182, f=w164) -> (s? t:f=w184:u32)
        n87 = Multiply(x=w181, y=w180) -> (x*y=w175:u32)
        n88 = Select(t=w175, s=w179, f=u32 0 ("Total_Rec")) -> (s? t:f=w189:u32)
        n89 = Multiply(x=w184, y=w186) -> (x*y=w187:u32)
        n90 = Bundle By Name(cluster=T4 {"Points Per A-Scan"=0, "A-Scans per B-Scan"=0, "Voltage Range"=4.0, "Card Resolution (bits)"=16} ("Imaging Parameters"), "Points Per A-Scan"=w170, "A-Scans per B-Scan"=w172, "Voltage Range"=sgl 4.0, "Card Resolution (bits)"=u16 16) -> (w171:T4)
        n91 = Bundle By Name(cluster=w168, "UseHeader"=u32 0, "Rec/Buffer"=w187, "Total_Rec"=w189) -> (w167:T5)
        n92 = local write "Async_Setting"(w167) -> ()
        n93 = local write "Imaging Parameters"(w171) -> ()
      }
      frame "Acquire Data", Default {
        # "Update and \nclear the \nEn Face"
        # "Tell the FFT the most\nup-to-date imaging\nparameters"
        n94 = Enqueue Element(queue=w213, element=OCT_Hardware_States."Initialize DAQ", error in (no error)=w212) -> (error out=w210:errorcluster)  [unwired: 1 in, 2 out]
        n95 = local read "Imaging Parameters"() -> (w236:T4)
        n96 = call "galvo_functional_global.vi"("State"=galvo_states."Run Raster", "error in (no error)"=w210) -> ("error out"=w227:errorcluster)  [unwired: 8 in, 1 out]
        n97 = local read "Async_Setting"() -> (w235:T5)
        n98 = call <vilib>:"Clear Errors.vi"("error in (no error)"=w227) -> ("error out"=w226:errorcluster)  [unwired: 5 in, 1 out]
        n99 = call "OCT Processing OpenCL.vi"("State"=processing_states."Update Imaging Parameters", "Input Parameters"=w236, "error in (no error)"=w226) -> ("error out"=w219:errorcluster)  [unwired: 8 in, 4 out]
        n100 = local read "Data Format"() -> (w238:T1)
        n101 = call "galvo_functional_global.vi"("State"=galvo_states."Get Scan Parameters", "error in (no error)"=w219) -> ("error out"=w220:errorcluster, "Scanning Output"=w228:T27)  [unwired: 8 in]
        n102 = call "Quick NPT Config.vi"("error in (no error)"=w210, "Data Format"=w238, "Async_Setting"=w235, "Value"=w231) -> ("error out"=w216:errorcluster, "Device Out"=w241:i32, 3:w221)  [unwired: 4 in]
        n103 = call "En Face Functional Global.vi"(7:En_Face_States."Clear En Face" ("En Face States"), "Error In"=w220, 9:w228) -> ("Error Out"=w218:errorcluster)  [unwired: 7 in, 1 out]
        n104 = Merge Errors(w216, w218) -> (w217:errorcluster)
        n105 = local read "Data Format"() -> (w215:T1)
        n106 = local read "Display"() -> (w214:T2)
        n107 = call "OCT Processing OpenCL.vi"("State"=processing_states."Get Queue", "error in (no error)"=w217) -> ("queue out"=w233:refnum<queue>, "error out"=w225:errorcluster)  [unwired: 9 in, 3 out]
        n108 = while {
          tunnel: w241 -> [w263]
          shift-right: [ATS_Async_Ctrl."Get" ("ATS_Async_Ctrl")] -> _
          shift-left: ATS_Async_Ctrl."StartCapture" ("ATS_Async_Ctrl") -> [w262]
          tunnel: w233 -> [w258]
          tunnel: [w257] -> w232
          tunnel: w221 -> [w256]
          tunnel: w225 -> [w252]
          tunnel: [w252] -> w224
          tunnel: w215 -> [w251]
          tunnel: w214 -> [w250]
          stop <- w257 stop-if-true
          n109 = call "ATS_AsyncDMA_Device.vi"("DeviceIn"=w263, "ATS_Async_Ctrl"=w262) -> ("Buffer"=w260:u16[], "Async_Status"=w255:T38)  [unwired: 9 in, 3 out]
          n110 = local read "Reset DAQ"() -> (w259:bool)
          n111 = call "DAQ Status.vi"("Enum"=DAQ_Status_States."Get", "Async_Status"=w255) -> ("DAQ Error?"=w253:bool, "Valid"=w254:bool)  [unwired: 8 in]
          n112 = Compound Arithmetic op=OR(w253, w259) -> (w257:bool)
          n113 = case shown="True" w254 {
            tunnel: w260 -> [_ w268]
            tunnel: w258 -> [_ w270]
            tunnel: w256 -> [_ w267]
            tunnel: w251 -> [_ w265]
            tunnel: w250 -> [_ w264]
            frame False {
              # "Do nothing"
            }
            frame True {
              n114 = call "Display Raw Data.vi"("Display"=w264, "Enum"=Display_Raw_Data_states."Add Processed", "Data Format"=w265, "Length"=w267, "Raw Data In"=w268) -> ()  [unwired: 7 in]
              n115 = Enqueue Element(queue=w270, element=w268, timeout in ms (-1)=50) -> ()  [unwired: 1 in, 3 out]
            }
          }
        }
        n116 = while {
          tunnel: w232 -> [w248]
          tunnel: [w245] -> w223
          tunnel: w224 -> [w245]
          stop <- w242 stop-if-true
          n117 = local read "Processing Finished"() -> (w247:bool)
          n118 = Wait (ms)(milliseconds to wait=u32 25) -> ()  [unwired: 1 out]
          n119 = local read "Reset DAQ"() -> (w243:bool)
          n120 = And(x=w248, y=w247) -> (x .and. y?=w244:bool)
          n121 = Or(x=w244, y=w243) -> (x .or. y?=w242:bool)
        }
        n122 = call "galvo_functional_global.vi"("State"=galvo_states."Reset", "error in (no error)"=w223) -> ()  [unwired: 8 in, 2 out]
      }
      frame "Acquire Background" {
        # "Update and \nclear the \nEn Face"
        # "Tell the FFT the most\nup-to-date imaging\nparameters"
        n123 = local read "Imaging Parameters"() -> (w285:T4)
        n124 = call "galvo_functional_global.vi"("State"=galvo_states."Run Raster", "error in (no error)"=w272) -> ("error out"=w280:errorcluster)  [unwired: 8 in, 1 out]
        n125 = local read "Async_Setting"() -> (w284:T5)
        n126 = call <vilib>:"Clear Errors.vi"("error in (no error)"=w280) -> ("error out"=w279:errorcluster)  [unwired: 5 in, 1 out]
        n127 = call "OCT Processing OpenCL.vi"("State"=processing_states."Update Imaging Parameters", "Input Parameters"=w285, "error in (no error)"=w279) -> ("error out"=w278:errorcluster)  [unwired: 8 in, 4 out]
        n128 = local read "Data Format"() -> (w286:T1)
        n129 = call "galvo_functional_global.vi"("State"=galvo_states."Get Scan Parameters", "error in (no error)"=w278) -> ("error out"=w276:errorcluster)  [unwired: 8 in, 1 out]
        n130 = call "Quick NPT Config.vi"("error in (no error)"=w272, "Data Format"=w286, "Async_Setting"=w284, "Value"=w283) -> ("error out"=w277:errorcluster, "Device Out"=w289:i32)  [unwired: 5 in]
        n131 = Merge Errors(w277, w276) -> (w273:errorcluster)
        n132 = while {
          tunnel: w289 -> [w299]
          shift-right: [ATS_Async_Ctrl."Get" ("ATS_Async_Ctrl")] -> _
          shift-left: ATS_Async_Ctrl."StartCapture" ("ATS_Async_Ctrl") -> [w298]
          tunnel: w273 -> [w295]
          tunnel: [w295] -> w274
          stop <- w291 stop-if-true
          n133 = local read "Imaging Parameters"() -> (w292:T4)
          n134 = call "ATS_AsyncDMA_Device.vi"("DeviceIn"=w299, "ATS_Async_Ctrl"=w298) -> ("Buffer"=w293:u16[], "Async_Status"=w296:T38)  [unwired: 9 in, 3 out]
          n135 = call "DAQ Status.vi"("Enum"=DAQ_Status_States."Get", "Async_Status"=w296) -> ("Valid"=w294:bool)  [unwired: 8 in, 1 out]
          n136 = case shown="True" w294 {
            selector: w294 -> [_ w304]
            tunnel: w293 -> [_ w308]
            tunnel: w292 -> [_ w307]
            tunnel: [FALSE w304] -> w291
            frame False {
            }
            frame True {
              n137 = Unbundle By Name(w307) -> ("A-Scans per B-Scan"=w306:i32, "Points Per A-Scan"=w305:i32)
              n138 = Reshape Array(w308, w306, w305) -> (w302:u16[][])
              n139 = call "Average BScan.vi"("B-Scan In"=w302) -> ("Averaged BScan"=w301:dbl[])  [unwired: 10 in]
              n140 = call "OCT Processing OpenCL.vi"("State"=processing_states."Set Background", "Background"=w301) -> ()  [unwired: 9 in, 5 out]
            }
          }
        }
        n141 = Enqueue Element(queue=w271, element=OCT_Hardware_States."Set Resampling Array", error in (no error)=w274) -> ()  [unwired: 1 in, 3 out]
      }
      frame "Acquire Data" {
        # "Close files and set save \nstate to do nothing"
        # "Update and \nclear the \nEn Face"
        # "Tell the FFT the most\nup-to-date imaging\nparameters"
        n142 = local read "Imaging Parameters"() -> (w338:T4)
        n143 = call "galvo_functional_global.vi"("State"=galvo_states."Run Raster", "error in (no error)"=w326) -> ("error out"=w323:errorcluster)  [unwired: 8 in, 1 out]
        n144 = call <vilib>:"Clear Errors.vi"("error in (no error)"=w323) -> ("error out"=w343:errorcluster)  [unwired: 5 in, 1 out]
        n145 = call "OCT Processing OpenCL.vi"("State"=processing_states."Update Imaging Parameters", "Input Parameters"=w338, "error in (no error)"=w343) -> ("error out"=w312:errorcluster)  [unwired: 8 in, 4 out]
        n146 = call "Save Data Functional Global.vi"("States"=Saving_Data_States."Get Queue", "error in (no error)"=w343) -> ("error out"=w314:errorcluster, "Saving Queue Out"=w329:refnum<queue>)  [unwired: 6 in, 2 out]
        n147 = call "galvo_functional_global.vi"("State"=galvo_states."Get Scan Parameters", "error in (no error)"=w312) -> ("error out"=w313:errorcluster, "Scanning Output"=w324:T27)  [unwired: 8 in]
        n148 = local read "Async_Setting"() -> (w317:T5)
        n149 = local read "Data Format"() -> (w318:T1)
        n150 = call "En Face Functional Global.vi"(7:En_Face_States."Clear En Face" ("En Face States"), "Error In"=w313, 9:w324) -> ("Error Out"=w310:errorcluster)  [unwired: 7 in, 1 out]
        n151 = call "Quick NPT Config.vi"("error in (no error)"=w314, "Data Format"=w318, "Async_Setting"=w317, "Value"=w315) -> ("error out"=w309:errorcluster, "Device Out"=w316:i32)  [unwired: 5 in]
        n152 = Merge Errors(w309, w310) -> (w311:errorcluster)
        n153 = call "OCT Processing OpenCL.vi"("State"=processing_states."Get Queue", "error in (no error)"=w311) -> ("queue out"=w331:refnum<queue>, "error out"=w333:errorcluster)  [unwired: 9 in, 3 out]
        n154 = while {
          tunnel: w333 -> [_]
          tunnel: [w349] -> w320
          i -> [w348]
          stop <- w347 stop-if-true
          # "Saves data as long as data is being fed into the Queue,\notherwise it will time out and halt this loop."
          n155 = case shown="0" w348 {
            tunnel: [FALSE w355] -> w347
            tunnel: [_ w352] -> w349
            frame 0 {
              # "Wait for data to Q up"
              n156 = Wait (ms)(milliseconds to wait=u32 500) -> ()  [unwired: 1 out]
            }
            frame 1, Default {
              n157 = local read "Data Format"() -> (w358:T1)
              n158 = Wait (ms)(milliseconds to wait=u32 100) -> ()  [unwired: 1 out]
              n159 = call "Save Data Functional Global.vi"("States"=Saving_Data_States."Save Data", "Data Format"=w358) -> ("error out"=w353:errorcluster)  [unwired: 6 in, 3 out]
              n160 = call "Save Data Functional Global.vi"("States"=Saving_Data_States."Get Queue Size", "error in (no error)"=w353) -> ("error out"=w352:errorcluster, "# elements in queue"=w354:i32)  [unwired: 6 in, 2 out]
              n161 = Equal To 0?(x=w354) -> (x = 0?=w355:bool)
            }
          }
        }
        n162 = while {
          shift-right: [ATS_Async_Ctrl."Get" ("ATS_Async_Ctrl")] -> _
          shift-left: ATS_Async_Ctrl."StartCapture" ("ATS_Async_Ctrl") -> [w371]
          tunnel: w331 -> [w367]
          tunnel: w329 -> [w366]
          tunnel: w316 -> [w361]
          stop <- w365 stop-if-true
          n163 = call "ATS_AsyncDMA_Device.vi"("DeviceIn"=w361, "ATS_Async_Ctrl"=w371) -> ("Buffer"=w369:u16[], "Async_Status"=w364:T38)  [unwired: 9 in, 3 out]
          n164 = local read "Reset DAQ"() -> (w368:bool)
          n165 = call "DAQ Status.vi"("Enum"=DAQ_Status_States."Get", "Async_Status"=w364) -> ("DAQ Error?"=w362:bool, "Valid"=w363:bool)  [unwired: 8 in]
          n166 = Compound Arithmetic op=OR(w362, w368) -> (w365:bool)
          n167 = case shown="True" w363 {
            tunnel: w369 -> [_ w374]
            tunnel: w369 -> [_ w375]
            tunnel: w367 -> [_ w376]
            tunnel: w366 -> [_ w373]
            frame False {
              # "Do nothing"
            }
            frame True {
              w372 = 50 ("timeout in ms (-1)")
              n168 = Enqueue Element(queue=w373, element=w374, timeout in ms (-1)=w372) -> ()  [unwired: 1 in, 3 out]
              n169 = Enqueue Element(queue=w376, element=w375, timeout in ms (-1)=w372) -> ()  [unwired: 1 in, 3 out]
            }
          }
        }
        n170 = while {
          tunnel: [w345] -> w319
          tunnel: w320 -> [w345]
          stop <- w344 stop-if-true
          n171 = local read "Processing Finished"() -> (w344:bool)
          n172 = Wait (ms)(milliseconds to wait=u32 25) -> ()  [unwired: 1 out]
        }
        n173 = call "galvo_functional_global.vi"("State"=galvo_states."Reset", "error in (no error)"=w319) -> ("error out"=w322:errorcluster)  [unwired: 8 in, 1 out]
        n174 = call "Save Data Functional Global.vi"("States"=Saving_Data_States."Close Files", "error in (no error)"=w322) -> ("error out"=w337:errorcluster)  [unwired: 6 in, 3 out]
        n175 = call "Save Data Functional Global.vi"("States"=Saving_Data_States."Do Nothing" ("Save State"), "error in (no error)"=w337) -> ("error out"=w335:errorcluster)  [unwired: 6 in, 3 out]
        n176 = Enqueue Element(queue=w340, element=OCT_Hardware_States."Set Resampling Array", error in (no error)=w335) -> ()  [unwired: 1 in, 3 out]
      }
      frame "Set Clock" {
        n177 = Wait (ms)(milliseconds to wait=u32 10) -> ()  [unwired: 1 out]
      }
      frame "Stop" {
        n178 = Release Queue(queue=w392, error in (no error)=w391) -> (error out=w390:errorcluster)  [unwired: 1 in, 2 out]
        n179 = call "OCT Processing OpenCL.vi"("State"=processing_states."Shutdown", "error in (no error)"=w390) -> ("error out"=w389:errorcluster)  [unwired: 9 in, 4 out]
        n180 = call "Save Data Functional Global.vi"("States"=Saving_Data_States."Shutdown", "error in (no error)"=w389) -> ("error out"=w386:errorcluster)  [unwired: 6 in, 3 out]
        n181 = call "galvo_functional_global.vi"("State"=galvo_states."Shutdown", "error in (no error)"=w386) -> ("error out"=w383:errorcluster)  [unwired: 8 in, 1 out]
        n182 = call "OpenCL Functional Global.vi"("States"=OpenCL_States."Delete Memory", "Error In"=w383) -> ("Error Out"=w381:errorcluster)  [unwired: 6 in, 3 out]
        n183 = call "OpenCL Functional Global.vi"("States"=OpenCL_States."Delete", "Error In"=w381) -> ("Error Out"=w380:errorcluster)  [unwired: 6 in, 3 out]
        n184 = flat-sequence {
          tunnel: w380 -> [_]
          frame #0 {
            w396 = 0 ("DeviceIn")
            n185 = call "ATS_AsyncDMA_Device.vi"("DeviceIn"=w396, "ATS_Async_Ctrl"=ATS_Async_Ctrl."Stop") -> ("ReadSamples_Out"=w395:T30)  [unwired: 9 in, 4 out]
            n186 = call "ATS_AsyncDMA_Device.vi"("DeviceIn"=w396, "ATS_Async_Ctrl"=ATS_Async_Ctrl."Abort", "ReadSamples"=w395) -> ()  [unwired: 8 in, 5 out]
          }
          frame #1 {
            n187 = Stop(stop? (T)=TRUE) -> ()
          }
        }
      }
      frame "Update DAQ Parameters" {
        w401 = T15 12 items=["20mV", "40mV", "50mV", "80mV", "100mV", "200mV", "400mV", "500mV", "800mV", "1 V", "1.25 V", "2 V", "4 V", "5 V", "8 V", "10 V", "16 V", "20 V", "40 V", "HiFi"] ("Input B.Range")
        w404 = u32 18 items=["1 kS/s", "2 kS/s", "5 kS/s", "10 kS/s", "20 kS/s", "50 kS/s", "100 kS/s", "200 kS/s", "500 kS/s", "1 MS/s", "2 MS/s", "5 MS/s", "10 MS/s", "20 MS/s", "50 MS/s", "100 MS/s", "125 MS/s", "160 MS/s", "180 MS/s"] ("ClckRate")
        n188 = local read "Clock Length"() -> (w403:u32)
        n189 = call "ATS_Device.vi"("BoardToVerify"=w399, "ATS_Check"=ATS_Check_Ctrl."Verify Board", "DevCtrl"=Device_Ctrl."Initialize", "DeviceIn"=0 ("Device")) -> ("error out"=w406:errorcluster, "DeviceOut"=w411:i32)  [unwired: 1 in, 5 out]
        n190 = Bundle By Name(cluster=w398, "Record.Length"=w403, "Clock.ClckSource"=ClockSource."Internal", "Clock.ClckRate"=w404, "Input B.Range"=w401, "Input A.Impedance"=Impedance."50 ohms") -> (w402:T7)
        n191 = call "ATS_Device.vi"("error in (no error)"=w406, "DevCtrl"=Device_Ctrl."Abort", "DeviceIn"=w411) -> ("DeviceOut"=w409:i32)  [unwired: 2 in, 6 out]
        n192 = call "ATS_MS_Set_Device.vi"("Set_Manually (F)"=FALSE, "Setup_In"=w402, "DeviceIn"=w409) -> ()  [unwired: 3 in, 6 out]
      }
      frame "Set Resampling Array" {
      }
      frame "Update DAQ Parameters" {
        n193 = call "Configure Alazar Cluster.vi"(10:"ATS9462" ("Alazar Board")) -> (3:w416)  [unwired: 10 in]
        n194 = property class="Clust (strict)"(reference=w416) -> ("Value"=w415:T7)  [unwired: 1 in, 2 out]
      }
      frame "Background Subtraction" {
        n195 = Enqueue Element(queue=w430, element=OCT_Hardware_States."Update DAQ Parameters", error in (no error)=w429) -> (queue out=w418:refnum<queue>, error out=w427:errorcluster)  [unwired: 1 in, 1 out]
        n196 = call "Display Message to User"("error in (no error)"=w427) -> ("error out"=w420:errorcluster)  [unwired: 9 in, 1 out]
        n197 = call "galvo_functional_global.vi"("State"=galvo_states."Center Galvos", "error in (no error)"=w420) -> ("error out"=w419:errorcluster)  [unwired: 8 in, 1 out]
        n198 = Enqueue Element(queue=w418, element=OCT_Hardware_States."Set Resampling Array", error in (no error)=w419) -> (error out=w421:errorcluster)  [unwired: 1 in, 2 out]
        n199 = property on="Calibrate" class="Bool"(error in=w421, "Visible"=TRUE) -> (error out=w423:errorcluster)  [unwired: 1 in, 1 out]
        n200 = property on="Calibrate" class="Bool"(error in=w423, "Blinking"=TRUE) -> ()  [unwired: 1 in, 2 out]
      }
      frame "Background Subtraction" {
        n201 = call "Display Message to User2"("error in (no error)"=w437) -> ("error out"=w438:errorcluster)  [unwired: 9 in, 1 out]
        n202 = call "galvo_functional_global.vi"("State"=galvo_states."Center Galvos", "error in (no error)"=w438) -> ("error out"=w433:errorcluster)  [unwired: 8 in, 1 out]
        n203 = Enqueue Element(queue=w435, element=OCT_Hardware_States."Initialize DAQ", error in (no error)=w433) -> (queue out=w434:refnum<queue>, error out=w432:errorcluster)  [unwired: 1 in, 1 out]
        n204 = Enqueue Element(queue=w434, element=OCT_Hardware_States."Acquire Background", error in (no error)=w432) -> ()  [unwired: 1 in, 3 out]
      }
      frame "Initialize Laser" {
        n205 = call "galvo_functional_global.vi"("State"=galvo_states."Get Scan Parameters", "error in (no error)"=w455) -> ("error out"=w453:errorcluster, "Scanning Output"=w452:T27)  [unwired: 8 in]
        n206 = Unbundle By Name(w452) -> ("A(cluster)/B"=w449:u32)
        n207 = Unbundle By Name(w448) -> ("Record.Length"=w447:u32)
        n208 = local read "B-Scans Per Buffer"() -> (w446:i32)
        n209 = Bundle By Name(cluster=T37 {"Depth"=1, "Height"=1, "Width"=1} ("Dimension"), "Depth"=w446, "Height"=w449, "Width"=w447) -> (w442:T37)
        n210 = call "OpenCL Functional Global.vi"("States"=OpenCL_States."Get U16 Memory Dimension", "Error In"=w453) -> ("Error Out"=w443:errorcluster, "U16 Dimensions"=w445:T37)  [unwired: 6 in, 2 out]
        n211 = Not Equal?(x=w442, y=w445) -> (x != y?=w444:bool)
        n212 = case shown="True" w444 {
          tunnel: w443 -> [_ w457]
          tunnel: w442 -> [_ w456]
          frame False {
          }
          frame True {
            n213 = call "OpenCL Functional Global.vi"("States"=OpenCL_States."Allocate Memory", "Error In"=w457, "Dimension"=w456) -> ()  [unwired: 5 in, 4 out]
          }
        }
      }
      frame "Initialize Galvos" {
        n214 = call "OpenCL Functional Global.vi"("States"=OpenCL_States."Delete Memory", "Error In"=w461) -> ()  [unwired: 6 in, 4 out]
      }
    }
  }
  n215 = while {
    tunnel: w10 -> [w462]
    tunnel: w11 -> [w463]
    stop <- FALSE stop-if-true
    # "User Interface Loop"
    n216 = event shown="[6] \"Calibrate\": Value Change" {
      selector: w463 -> [_ _ _ _ _ _ _]
      dyn-events: _ -> [_ _ _ _ _ _ _]
      timeout: _ -> [_ _ _ _ _ _ _]
      tunnel: w462 -> [w470 w472 w483 _ w497 _ _]
      event User Event {
        n217 = event-data() -> ("Reset Galvos"=w471:bool)  [unwired: 1 in]
        n218 = local write "Reset DAQ"(w471) -> ()
        n219 = Enqueue Element(queue=w470, element=OCT_Hardware_States."Initialize Galvos") -> (queue out=w467:refnum<queue>)  [unwired: 2 in, 2 out]
        n220 = Enqueue Element(queue=w467, element=OCT_Hardware_States."Initialize Laser") -> (queue out=w465:refnum<queue>)  [unwired: 2 in, 2 out]
        n221 = Enqueue Element(queue=w465, element=OCT_Hardware_States."Initialize DAQ") -> ()  [unwired: 2 in, 3 out]
      }
      event "Stop Button": Value Change {
        n222 = event-data() -> ()  [unwired: 1 in, 1 out]
        n223 = flat-sequence {
          tunnel: w472 -> [w475]
          tunnel: [w475] -> w473
          tunnel: w473 -> [w480]
          frame #0 {
            w474 = TRUE ("Reset DAQ")
            n224 = local write "Processing Finished"(w474) -> ()
            n225 = local write "Reset DAQ"(w474) -> ()
          }
          frame #1 {
            n226 = Enqueue Element(queue=w480, element=OCT_Hardware_States."Set Resampling Array") -> (queue out=w477:refnum<queue>, error out=w478:errorcluster)  [unwired: 2 in, 1 out]
            n227 = Enqueue Element(queue=w477, element=OCT_Hardware_States."Stop", error in (no error)=w478) -> ()  [unwired: 1 in, 3 out]
          }
        }
      }
      event "Save Sweep": Value Change {
        n228 = event-data() -> ()  [unwired: 1 in, 1 out]
        n229 = flat-sequence {
          tunnel: [w484] -> w482
          tunnel: w482 -> [w490]
          tunnel: [w488] -> w481
          tunnel: w483 -> [w492]
          tunnel: w481 -> [_]
          frame #0 {
            n230 = call "File Dialog2"("prompt"="Select Path for saving") -> ("selected path"=w484:path)  [unwired: 11 in, 3 out]
          }
          frame #1 {
            n231 = local read "Imaging Parameters"() -> (w487:T4)
            n232 = local write "Save Data"(TRUE ("Save Data")) -> ()
            n233 = call "Save Data Functional Global.vi"("Input Parameters"=w487, "States"=Saving_Data_States."Create Files", "Folder"=w490) -> ("error out"=w488:errorcluster)  [unwired: 5 in, 3 out]
          }
          frame #2 {
            n234 = Enqueue Element(queue=w492, element=OCT_Hardware_States."Set Resampling Array") -> ()  [unwired: 2 in, 3 out]
          }
          frame #3 {
            n235 = local write "Reset DAQ"(TRUE ("Reset DAQ")) -> ()
          }
        }
      }
      event User Event {
        n236 = event-data() -> ()  [unwired: 1 in, 1 out]
        n237 = call "OCT Processing OpenCL.vi"("State"=processing_states."Get Size") -> ("# elements in queue"=w495:i32)  [unwired: 10 in, 4 out]
        n238 = Equal To 0?(x=w495) -> (x = 0?=→"Processing Finished":bool)
      }
      event Menu Selection (User) {
        n239 = event-data() -> ("ItemTag"=w498:string)  [unwired: 1 in, 2 out]
        n240 = case shown="\"DAQ Status\"" w498 {
          tunnel: w497 -> [_ _ w502 _ _ w514 w518 _]
          frame "Raw Data", Default {
            n241 = call "Display Raw Data.vi"("Enum"=Display_Raw_Data_states."Show") -> ()  [unwired: 11 in]
          }
          frame "DAQ Status" {
            n242 = call "DAQ Status.vi"("Enum"=DAQ_Status_States."Show") -> ()  [unwired: 9 in, 2 out]
          }
          frame "Configure_DAQ" {
            n243 = flat-sequence {
              tunnel: w502 -> [w508]
              tunnel: [w508] -> w501
              frame #0 {
                n244 = local write "Reset DAQ"(TRUE ("Reset DAQ")) -> ()
              }
            }
            n245 = Enqueue Element(queue=w501, element=OCT_Hardware_States."Set Resampling Array") -> (queue out=w504:refnum<queue>, error out=w505:errorcluster)  [unwired: 2 in, 1 out]
            n246 = Enqueue Element(queue=w504, element=OCT_Hardware_States."Update DAQ Parameters", error in (no error)=w505) -> ()  [unwired: 1 in, 3 out]
          }
          frame "En Face" {
            n247 = call "En Face Functional Global.vi"(7:En_Face_States."Show" ("En Face States")) -> ()  [unwired: 9 in, 2 out]
          }
          frame "Save Sweep" {
            n248 = property on="Save Sweep" class="Bool (strict)"("Val(Sgnl)"=TRUE ("Value (Signaling)")) -> ()  [unwired: 2 in, 2 out]
          }
          frame "K-Space Correction" {
            n249 = Enqueue Element(queue=w514, element=OCT_Hardware_States."Background Subtraction") -> (error out=w512:errorcluster)  [unwired: 2 in, 2 out]
            n250 = flat-sequence {
              tunnel: w512 -> [_]
              tunnel: [TRUE] -> w511
              frame #0 {
              }
            }
            n251 = local write "Reset DAQ"(w511) -> ()
          }
          frame "Background Subtraction" {
            n252 = Enqueue Element(queue=w518, element=OCT_Hardware_States."Background Subtraction") -> (error out=w517:errorcluster)  [unwired: 2 in, 2 out]
            n253 = flat-sequence {
              tunnel: [w521] -> _
              tunnel: w517 -> [w521]
              tunnel: [TRUE ("Reset DAQ")] -> w516
              frame #0 {
              }
            }
            n254 = local write "Reset DAQ"(w516) -> ()
          }
          frame "Configure_Galvos" {
            n255 = call "galvo_functional_global.vi"("State"=galvo_states."Show") -> ()  [unwired: 9 in, 2 out]
          }
        }
      }
      event "Save Sweep Button": Value Change {
        n256 = event-data() -> ()  [unwired: 1 in, 1 out]
        n257 = property on="Save Sweep" class="Bool (strict)"("Val(Sgnl)"=TRUE ("Value (Signaling)")) -> ()  [unwired: 2 in, 2 out]
      }
      event "Calibrate": Value Change {
        n258 = event-data() -> ()  [unwired: 1 in, 1 out]
        n259 = property on="Calibrate" class="Bool"("Visible"=FALSE) -> (error out=w528:errorcluster)  [unwired: 2 in, 1 out]
        n260 = property on="Calibrate" class="Bool"(error in=w528, "Blinking"=FALSE) -> ()  [unwired: 1 in, 2 out]
        n261 = call "Clock Frequency generator hilbert without wavepond.vi"("k-space signal in"=u16[] array[5000 elements]) -> ("Zero Crossing Resample Index"=w525:i32[])  [unwired: 10 in]
        n262 = call "OCT Processing OpenCL.vi"("State"=processing_states."Set Reample Array", "Resample Array"=w525) -> ()  [unwired: 9 in, 5 out]
      }
    }
  }
  n263 = while {
    stop <- w532 stop-if-true
    # "Display Loop"
    # "Sometimes a timeout event sends\na 0 array, this stops the flickering\nof the front panl due to those \ntimeout events"
    # "This takes the 0th element of the processed data,\nthe other elements will NOT be displayed"
    # "This loop just gets the last b-scan processed wheter in real time mode or not. \nJust meant to update the front panel Asynchronously.  This frame is NOT\nguarenteed to view every BScan, just the last one processed."
    n264 = call "OCT Processing OpenCL.vi"("State"=processing_states."Get Last Processed BScan") -> ("Processed OCT Data"=w537:T28, "error out"=w530:errorcluster)  [unwired: 10 in, 3 out]
    n265 = case shown="\"Channel B\"" "Display" {
      tunnel: w537 -> [w544 w545]
      tunnel: [w542 w546] -> w535
      frame "Channel A", Default {
        n266 = Unbundle By Name(w544) -> ("Intensity A"=w543:sgl[][][])
        n267 = Index Array(array=w543) -> (element=w542:sgl[][])  [unwired: 3 in]
      }
      frame "Channel B" {
        n268 = Unbundle By Name(w545) -> ("Intensity B"=w547:sgl[][][])
        n269 = Index Array(array=w547) -> (element=w546:sgl[][])  [unwired: 3 in]
      }
    }
    n270 = Array Size(array=w535) -> (size(s)=w536:i32[])
    n271 = Multiply Array Elements(1:w536) -> (0:w534:i32)
    n272 = Equal To 0?(x=w534) -> (x = 0?=w533:bool)
    n273 = case shown="False" w533 {
      tunnel: w535 -> [w540 _]
      frame False {
        "BScan" <- w540
      }
      frame True {
        n274 = Wait Until Next ms Multiple(millisecond multiple=u32 10) -> ()  [unwired: 1 out]
      }
    }
    n275 = local read "Stop Button"() -> (w531:bool)
    n276 = Or(x=w531, y=w530) -> (x .or. y?=w532:bool)
  }
